vi "Map Find.vi"(8 "Error In":errorcluster) -> (0 "Error Out":errorcluster)   [LabVIEW 2018, in "Tests.lvlib" / "Data.lvlib"]
uses:
  Data.lvlib
  src/Toolkit/Data/String/String.lvclass
  src/Toolkit/Data/Type Defintions/Types.ctl
  src/Toolkit/Data/String/String.lvclass/String.ctl
  src/Toolkit/Data/Pair/Pair.lvclass
  D:/Users/cfield/Code/Field R&D Services/Labstache/src/Toolkit/Data/Datum/Datum.lvclass
  src/Toolkit/Data/Array/Array.lvclass
  src/Toolkit/Data/Pair/Support/From String.vi
  src/Toolkit/Data/Array/Support/From Data.vi
  src/Toolkit/Data/Pair/Support/From Datum.vi
  src/Toolkit/Data/Map/Support/From Pair Array.vi
  src/Toolkit/Data/Datum/Datum.lvclass
  <vilib>/addons/_JKI Toolkits/Caraya/classes/Test/Test.lvclass
  <vilib>/addons/_JKI Toolkits/Caraya/classes/Assert/Assert.lvclass
  src/Toolkit/Data/Map/Map.lvclass
  src/Toolkit/Data/Data.lvlib
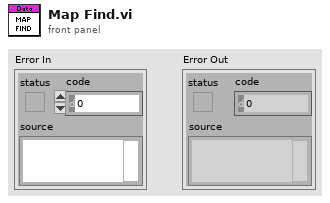
[diagram p1: front panel]
types:
  T1 = typedef "Toolkit.lvlib/Data.lvlib/Types.ctl" = enum16{"Array", "Boolean", "Function", "Map", "Null", "Pair", "Path", "String", "Unknown"}
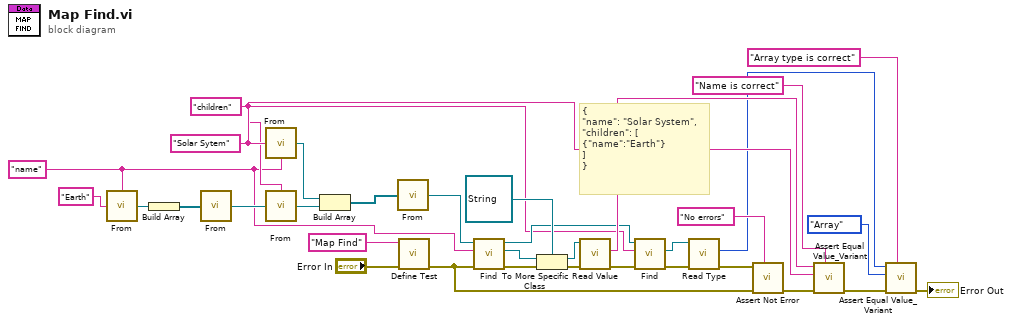
[diagram p0: block diagram]
diagram:
  w10 = "children" ("Key")
  w9 = "name" ("Key")
  w13 = "Solar Sytem" ("Value")
  # "{\n\"name\": \"Solar System\",\n\"children\": [\n{\"name\":\"Earth\"}\n]\n}"
  n1 = call-poly "From.vi"("Value"="Earth", "Key"=w9) -> ("Pair"=w27:refnum<class "Pair.lvclass">)
  n2 = Build Array(w27) -> (w26:refnum<class "Pair.lvclass">[])
  n3 = call-poly "From.vi"("Data"=w26) -> ("Array"=w25:refnum<class "Array.lvclass">)  [unwired: 1 in]
  n4 = call-poly "From.vi"("Value"=w13, "Key"=w9) -> ("Pair"=w19:refnum<class "Pair.lvclass">)
  n5 = call-poly "From.vi"("Value"=w25, "Key"=w10) -> ("Pair"=w24:refnum<class "Pair.lvclass">)
  n6 = Build Array(w19, w24) -> (w23:refnum<class "Pair.lvclass">[])
  n7 = call-poly "From.vi"("Pairs"=w23) -> ("Map"=w22:refnum<class "Map.lvclass">)  [unwired: 1 in]
  n8 = call <vilib>:"Define Test.vi"("error in (no error)"="Error In", "Label (VI Title)"="Map Find") -> ("error out"=w21:errorcluster)  [unwired: 9 in]
  n9 = call "Find.vi"("Error In"=w21, "Key"=w9, "Map In"=w22) -> ("Error Out"=w20:errorcluster, "Value"=w18:refnum<class "Datum.lvclass">, "Map Out"=w11:refnum<class "Map.lvclass">)  [unwired: 5 in, 1 out]
  n10 = To More Specific Class(target class=refnum<class "String.lvclass"> refnum ("Toolkit.lvlib:Data.lvlib:String.lvclass"), reference=w18, error in=w20) -> (specific class reference=w15:refnum<class "String.lvclass">, error out=w16:errorcluster)
  n11 = call "Read Value.vi"("Error In"=w16, "String In"=w15) -> ("Error Out"=w12:errorcluster, "Value"=w14:string)  [unwired: 7 in, 1 out]
  n12 = call "Find.vi"("Error In"=w12, "Key"=w10, "Map In"=w11) -> ("Error Out"=w7:errorcluster, "Value"=w8:refnum<class "Datum.lvclass">)  [unwired: 5 in, 2 out]
  n13 = call-dynamic "Read Type.vi"("Error In"=w7, "Datum In"=w8) -> ("Error Out"=w6:errorcluster, "Type"=w3:T1)  [unwired: 7 in, 1 out]
  n14 = call <vilib>:"Assert Not Error.vi"("Label"="No errors", "error in (no error)"=w21, "Not Error?"=w6) -> ("error out"=w30:errorcluster)  [unwired: 8 in]
  n15 = call <vilib>:"Assert Equal Value_Variant.vi"("Label"="Name is correct", "error in (no error)"=w30, "Y"=w13, "X"=w14) -> ("error out"=w5:errorcluster)  [unwired: 7 in]
  n16 = call <vilib>:"Assert Equal Value_Variant.vi"("Label"="Array type is correct", "error in (no error)"=w5, "Y"=Types."Array" ("Type"), "X"=w3) -> ("error out"=→"Error Out":errorcluster)  [unwired: 7 in]
